vi "Change menu button color as per screen index.vi"(8 "error in (no error)":errorcluster, 10 "Screen Index":i32, 11 "Array":refnum<vi>[](array[refnum])) -> (0 "error out":errorcluster)   [LabVIEW 2017]
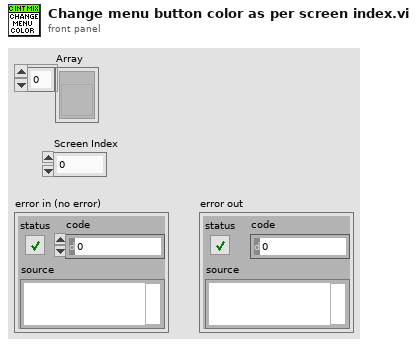
[diagram p1: front panel]
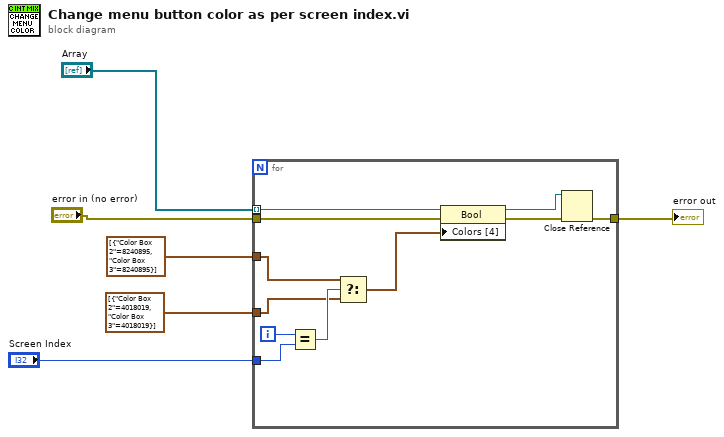
[diagram p0: block diagram]
diagram:
  n1 = for {
    tunnel: "Array" -> [w12] mode=indexing
    tunnel: cluster{"Color Box 2":u32, "Color Box 3":u32}[] [{"Color Box 2"=8240895, "Color Box 3"=8240895}] ("Colors [4]") -> [w13]
    tunnel: cluster{"Color Box 2":u32, "Color Box 3":u32}[] [{"Color Box 2"=4018019, "Color Box 3"=4018019}] ("Colors [4]") -> [w14]
    tunnel: "Screen Index" -> [w16]
    tunnel: [w7] -> w6
    tunnel: "error in (no error)" -> [w10]
    i -> [w17]
    n2 = Equal?(x=w17, y=w16) -> (x = y?=w15:bool)
    n3 = Select(t=w13, s=w15, f=w14) -> (s? t:f=w11:cluster{"Color Box 2":u32, "Color Box 3":u32}[])
    n4 = property class="Bool"(reference=w12, error in=w10, "Colors [4]"=w11) -> (reference out=w9:refnum<vi>, error out=w8:errorcluster)
    n5 = Close Reference(reference=w9, error in (no error)=w8) -> (error out=w7:errorcluster)
  }
  "error out" <- w6
